vi "Oil_Refinery.vi"() -> ()   [LabVIEW 2024]
uses:
  <vilib>/addons/control/pid/pid.llb/PID (DBL).vi
  <vilib>/addons/control/pid/NI_PID_pid.lvlib
panel:
  out "POWER (W)":dbl(knob) scale=0.0..100000.0 scale format="%#.2f"
  out "U_OUT":dbl(knob) scale=0.0..10000.0
  out "U_IN":dbl(knob) scale=0.0..120000.0
  out "Transformer_On_Light":bool
  in  "Transformer_On":bool
  out "Res Debit":dbl format="%#.2g"
  out "Dis Debit":dbl format="%#.2g"
  out "Gas Debit":dbl format="%#.2g"
  out "Crude Oil Debit":dbl(knob) scale=0.0..10.0
  out "PressPipe3":bool
  in  "EMPTY\nBOILER":bool
  in  "Graph Monitor":T1(tab)
  out "BOILER TEMPERATURE":dbl(graph)=35.0
  out "PID OUTPUT":dbl(graph)
  out "PID-TEMP TREND":cluster{dbl[], dbl[]}(graph)={[35.0, 35.0, 35.0, 35.0, 35.0, 35.0, 35.0, 35.0, 35.0, 35.0, 35.0, 35.0, 35.0, 35.0, 35.0, 35.0, 35.0, 35.0, 35.0, 35.0, 35.0, 35.0, 35.0, 35.0, 35.0, 35.0, 35.0, 35.0, 35.0, 35.0, 35.0, 35.0, 35.0, 35.0, 35.0, 35.0], [35.0, 35.0, 35.0, 35.0, 35.0, 35.0, 35.0, 35.0, 35.0, 35.0, 35.0, 35.0, 35.0, 35.0, 35.0, 35.0, 35.0, 35.0, 35.0, 35.0, 35.0, 35.0, 35.0, 35.0, 35.0, 35.0, 35.0, 35.0, 35.0, 35.0, 35.0, 35.0, 35.0, 35.0, 35.0, 35.0]}
  in  "PID gains":T2={"proportional gain (Kc)"=2.0, "integral time (Ti, min)"=0.05, "derivative time (Td, min)"=0.1}
  in  "HEATER POWER":u64(knob) scale=0.0..10.0
  out "PID output":dbl format="%.2f"
  out "PID %":dbl(slide)=35.0 scale=0.0..100.0 scale format="%#.2g"
  out "BAR":dbl(knob)=0.8301077246178509 scale=0.0..100.0
  out "HEATER":bool
  out "BOILER TEMP":dbl(knob)=35.0 scale=0.0..800.0
  out "RESIDUE":dbl(slide) scale=0.0..100.0
  out "DIESEL":dbl(slide) scale=0.0..100.0
  out "GASOLINE":dbl(slide) scale=0.0..100.0
  out "BOILER":dbl(slide) scale=0.0..100.0
  in  "Setpoint °C":dbl(knob)=100.0 scale=100.0..800.0
  in  "EMPTY\nCRUDE\nOIL \nTANK":bool
  out "Boiler Level":dbl(knob) scale=0.0..100.0 scale format="%#.2g"
  out "?":bool
  in  "Refill\nCrude Oil\nTank":bool
  out "Crude Oil Level":dbl(knob) scale=0.0..100.0 scale format="%#.2g"
  out "?":bool
  out "?":bool
  out "?":bool
  out "?":bool
  out "?":bool
  out "?":bool
  out "?":bool
  in  "Over\nPressure\nValve":bool
  in  "OIL PUMP":bool
  in  "Residue \nValve":bool
  in  "Diesel\nValve":bool
  in  "Gasoline Valve":bool
  in  "Crude \nOil\nValve":bool
  in  "STOP SIM":bool
  in  "HEATER":bool
  out "GaspolinePipe2":bool
  out "DieselPipe2":bool
  out "ResiduePipe2":bool
  out "OilPipe2":bool
  out "PressPipe2":bool
  out "PressPipe1":bool
  out "GaspolinePipe1":bool
  out "DieselPipe1":bool
  out "ResiduePipe1":bool
  out "OilPipe3":bool
  out "BOILER PRESSURE":dbl(slide) scale=0.0..100.0
  out "Oil_Pump":bool
  out "OilPipe1":bool
  out "Residue_Valve":bool
  out "Diesel_Valve":bool
  out "Gasoline_Valve":bool
  out "OverPressure_Valve":bool
  out "Crude_Oil_Valve":bool
  out "Alarm and Event Display":refnum<k7>(container)
  in  "Set Crude Oil Level":dbl(slide) scale=0.0..100.0
  out "CRUDE OIL TANK":dbl(slide) scale=0.0..100.0
  # "GREASY DUCK\n OIL PLANT"
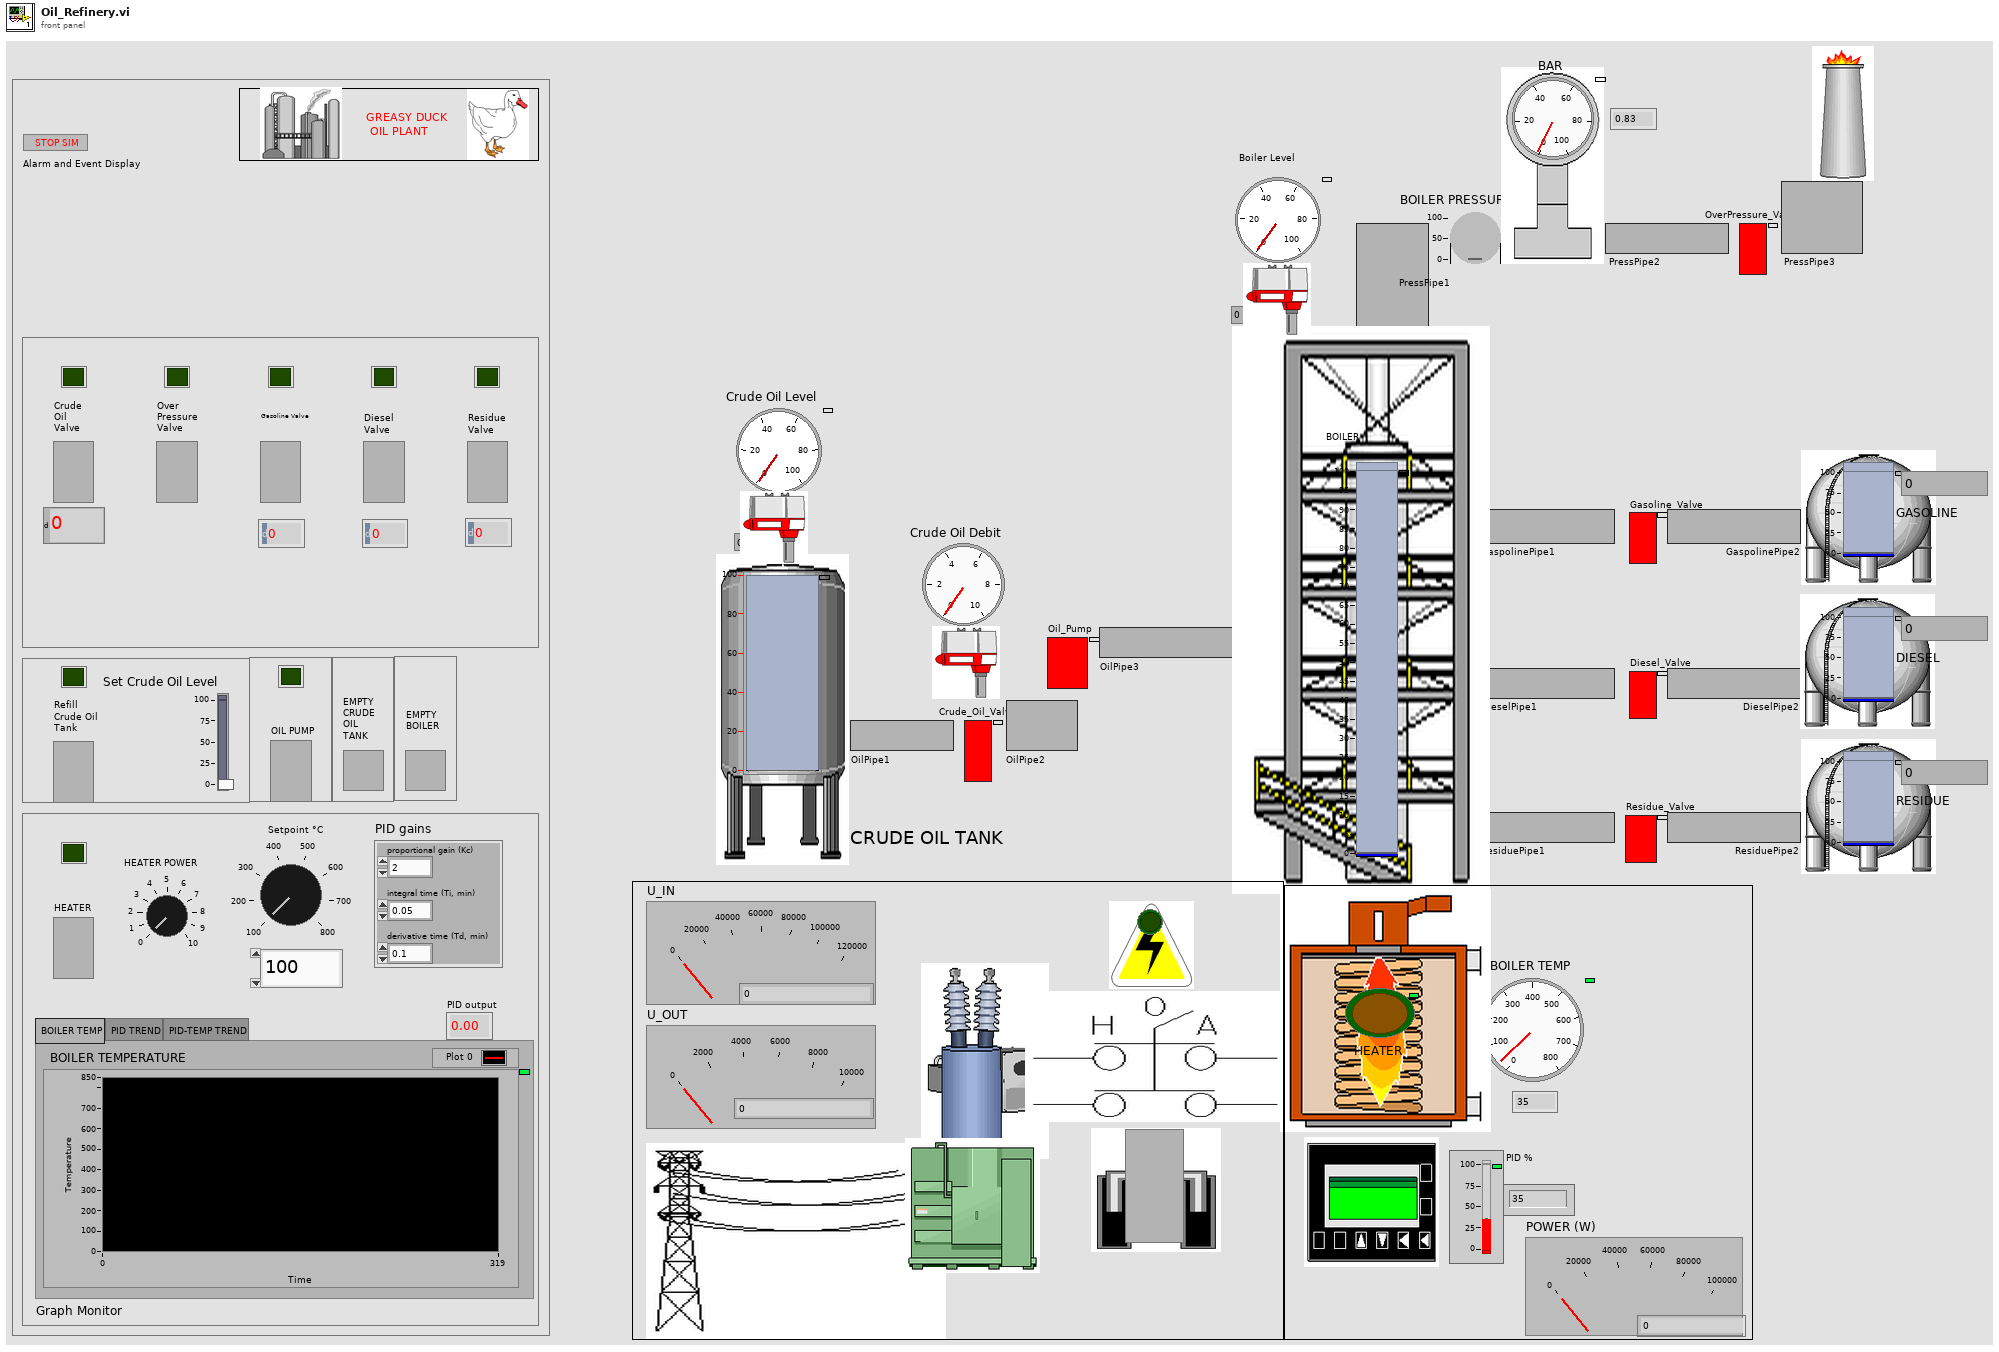
[diagram p1: front panel]
types:
  T1 = enum32{"BOILER TEMP", "PID TREND", "PID-TEMP TREND"}
  T2 = cluster{"proportional gain (Kc)":dbl, "integral time (Ti, min)":dbl, "derivative time (Td, min)":dbl}
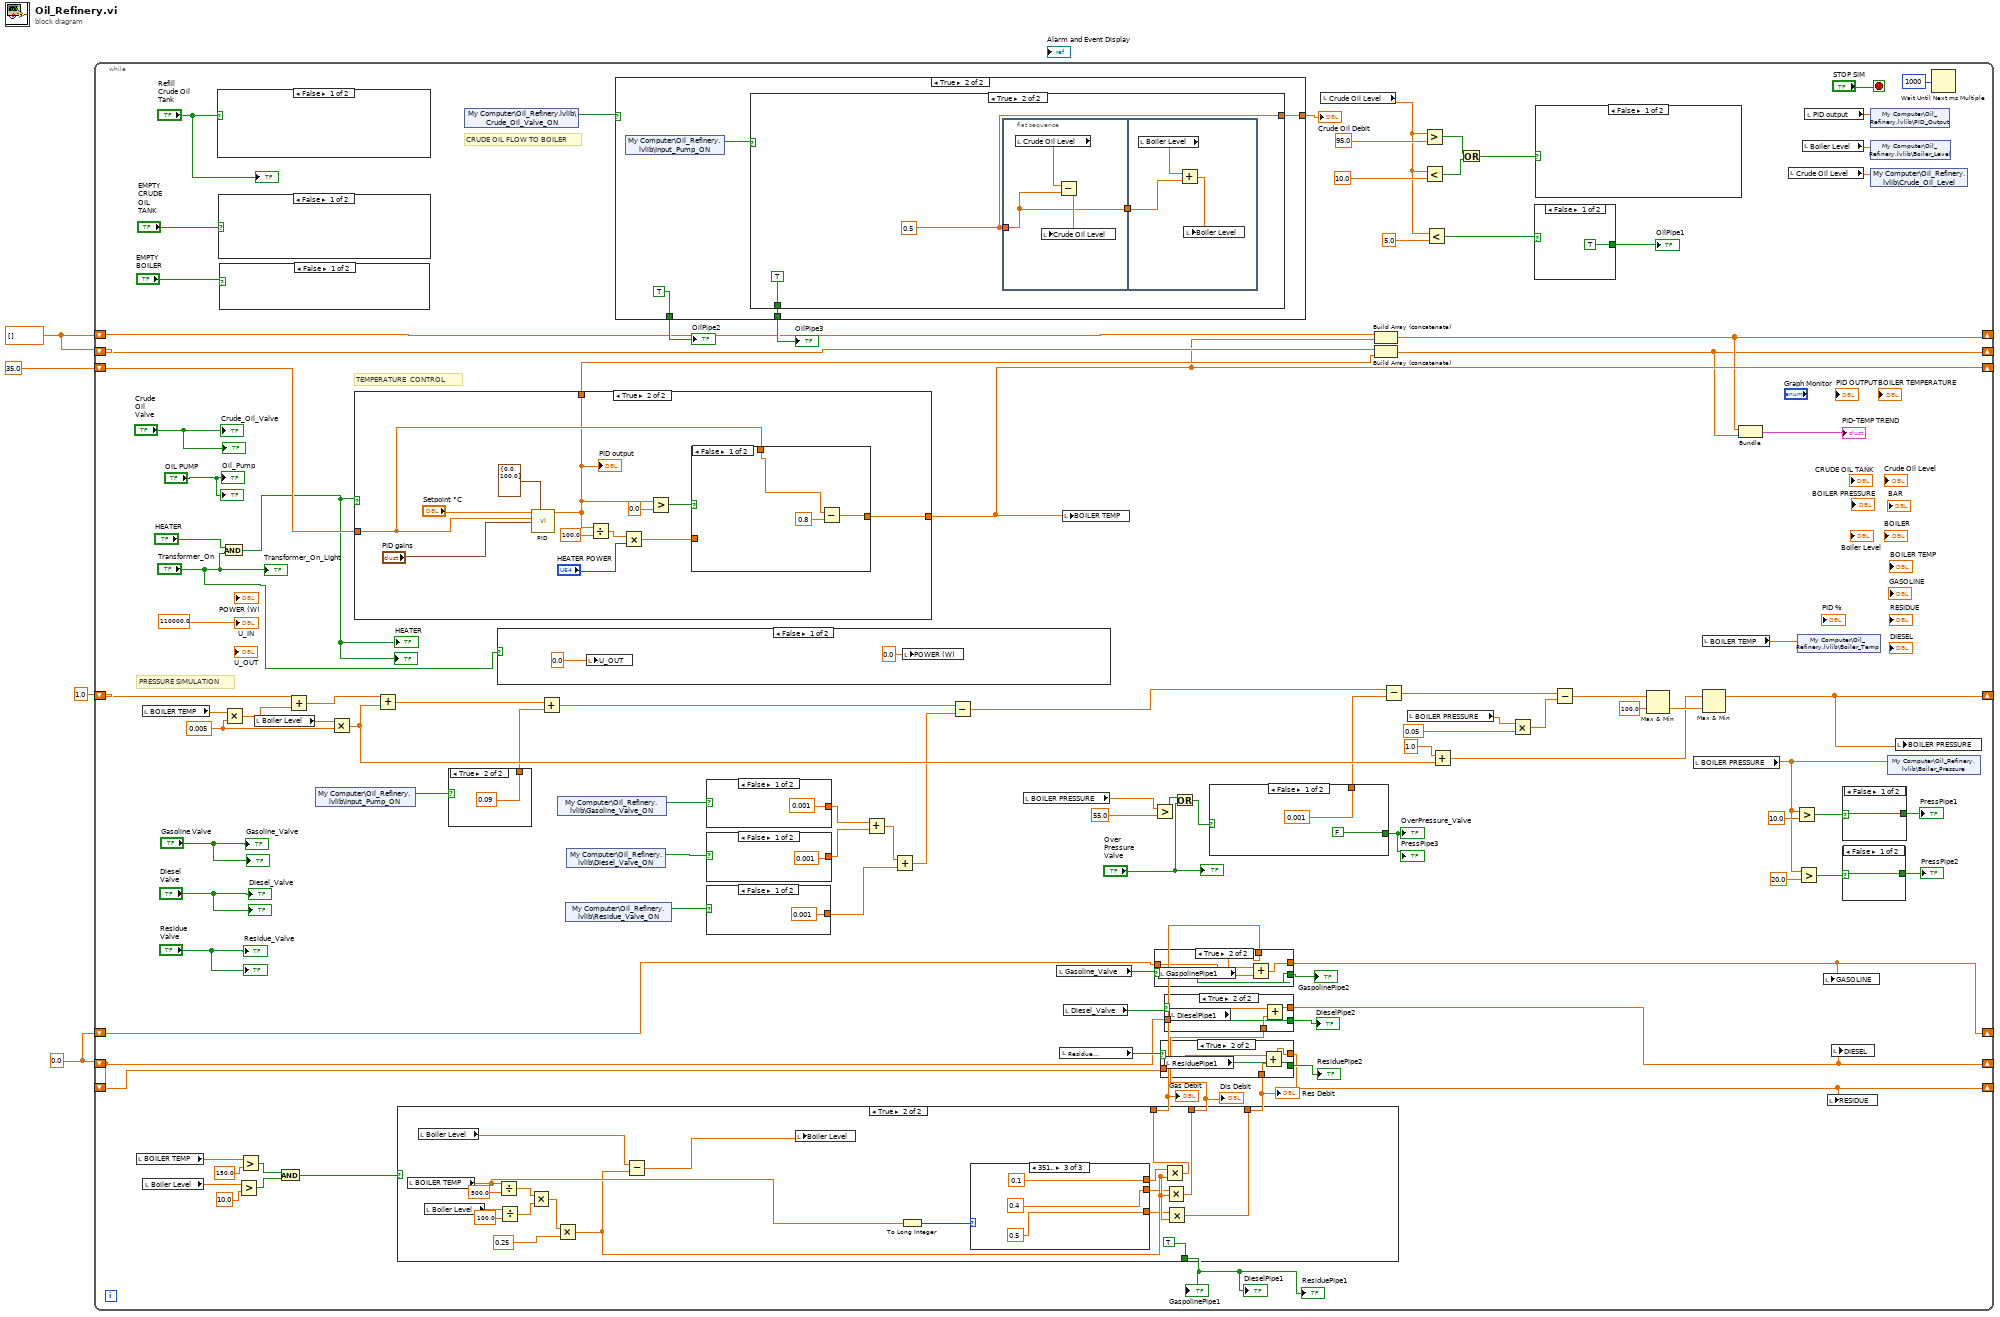
[diagram p0: block diagram]
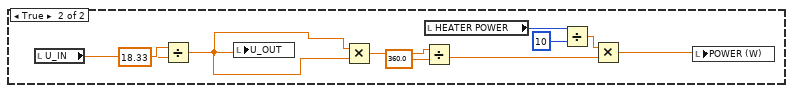
[diagram p2: hidden frame]
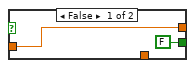
[diagram p3: hidden frame]
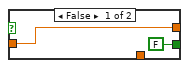
[diagram p4: hidden frame]
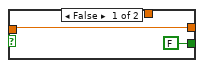
[diagram p5: hidden frame]
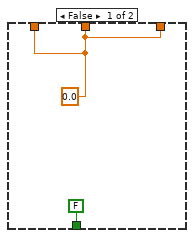
[diagram p6: hidden frame]
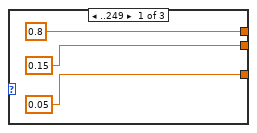
[diagram p7: hidden frame]
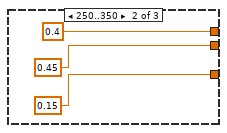
[diagram p8: hidden frame]
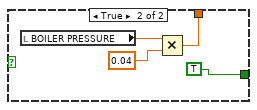
[diagram p11: hidden frame]
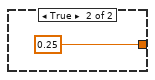
[diagram p12: hidden frame]
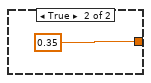
[diagram p13: hidden frame]
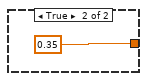
[diagram p14: hidden frame]
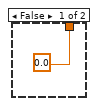
[diagram p15: hidden frame]
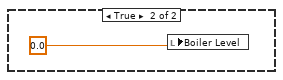
[diagram p16: hidden frame]
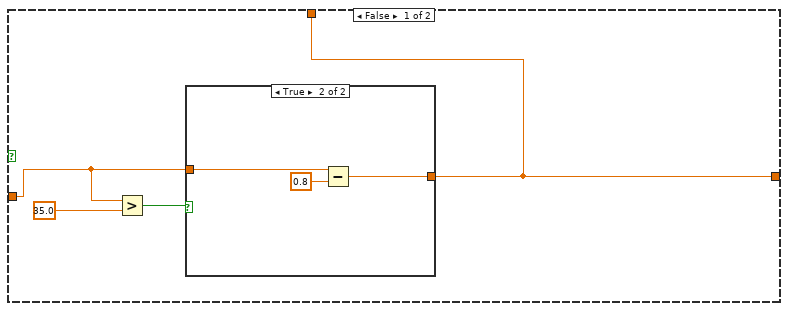
[diagram p17: hidden frame]
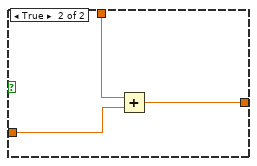
[diagram p19: hidden frame]
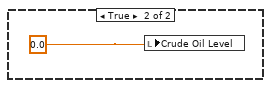
[diagram p20: hidden frame]
diagram:
  w1 = 0.0
  w3 = dbl[] []
  n1 = while {
    shift-right: [w82] -> _
    shift-left: 35.0 -> [w88]
    shift-right: [w80] -> _
    shift-left: w3 -> [w85]
    shift-right: [w79] -> _
    shift-left: w3 -> [w84]
    shift-right: [w71] -> _
    shift-left: 1.0 -> [w76]
    shift-right: [w10] -> _
    shift-left: w1 -> [w13]
    shift-right: [w11] -> _
    shift-left: w1 -> [w18]
    shift-right: [w12] -> _
    shift-left: w1 -> [w17]
    stop <- "STOP SIM" stop-if-true
    w65 = 0.005
    # "CRUDE OIL FLOW TO BOILER"
    # "TEMPERATURE  CONTROL"
    # "PRESSURE SIMULATION"
    n2 = local read "BOILER TEMP"() -> (w32:dbl)
    n3 = local read "BOILER TEMP"() -> (w74:dbl)
    n4 = local read "Boiler Level"() -> (w31:dbl)
    n5 = case shown="False" "Refill\nCrude Oil\nTank" {
      frame False {
      }
      frame True {
        n6 = local write "Crude Oil Level"("Set Crude Oil Level") -> ()
      }
    }
    n7 = case shown="False" "EMPTY\nCRUDE\nOIL \nTANK" {
      frame False {
      }
      frame True {
        n8 = local write "Crude Oil Level"(0.0) -> ()
      }
    }
    n9 = case shown="False" "EMPTY\nBOILER" {
      frame False {
      }
      frame True {
        n10 = local write "Boiler Level"(0.0) -> ()
      }
    }
    n11 = And(x="HEATER", y="Transformer_On") -> (x .and. y?=w7:bool)
    "?" <- w7
    "HEATER" <- w7
    n12 = Multiply(x=w74, y=w65) -> (x*y=w75:dbl)
    n13 = Greater?(x=w31, y=10.0) -> (0:w27:bool)
    n14 = Greater?(x=w32, y=150.0) -> (0:w28:bool)
    n15 = local read "Boiler Level"() -> (w64:dbl)
    n16 = And(x=w28, y=w27) -> (x .and. y?=w26:bool)
    n17 = Add(x=w76, y=w75) -> (x+y=w66:dbl)
    n18 = shared-variable "My Computer\\Oil_Refinery.lvlib\\Input_Pump_ON"() -> (w60:bool)  [unwired: 1 in, 1 out]
    n19 = Multiply(x=w64, y=w65) -> (x*y=w61:dbl)
    n20 = case shown="True" w7 {
      tunnel: w88 -> [w192 w201]
      tunnel: [w190 w203] -> w82
      tunnel: [w190 w198] -> w83
      frame False {
        n21 = Greater?(x=w192, y=35.0) -> (0:w193:bool)
        n22 = case shown="True" w193 {
          tunnel: [w194 w197] -> w190
          tunnel: w192 -> [w194 w196]
          frame False {
          }
          frame True {
            n23 = Subtract(x=w196, y=0.8) -> (x-y=w197:dbl)
          }
        }
      }
      frame True {
        n24 = call-poly <vilib>:"PID.vi"("output range"=cluster{"output high":dbl, "output low":dbl} {"output high"=0.0, "output low"=100.0}, "PID gains"="PID gains", "process variable"=w201, "setpoint"="Setpoint °C") -> ("output"=w198:dbl)  [unwired: 6 in, 1 out]
        "PID output" <- w198
        n25 = Divide(x=w198, y=100.0) -> (x/y=w205:dbl)
        n26 = Multiply(x=w205, y="HEATER POWER") -> (x*y=w202:dbl)
        n27 = Greater?(x=w198, y=0.0) -> (0:w200:bool)
        n28 = case shown="False" w200 {
          tunnel: [w211 w215] -> w203
          tunnel: w202 -> [_ w214]
          tunnel: w201 -> [w210 w213]
          frame False {
            n29 = Subtract(x=w210, y=0.8) -> (x-y=w211:dbl)
          }
          frame True {
            n30 = Add(x=w213, y=w214) -> (x+y=w215:dbl)
          }
        }
      }
    }
    n31 = Add(x=w66, y=w61) -> (x+y=w59:dbl)
    n32 = case shown="True" w26 {
      tunnel: [FALSE TRUE] -> w25
      tunnel: [w141 w145] -> w16
      tunnel: [w141 w144] -> w15
      tunnel: [w141 w143] -> w14
      frame False {
        w141 = 0.0
      }
      frame True {
        n33 = local read "BOILER TEMP"() -> (w151:dbl)
        n34 = local read "Boiler Level"() -> (w154:dbl)
        n35 = local read "Boiler Level"() -> (w160:dbl)
        n36 = Divide(x=w151, y=500.0) -> (x/y=w158:dbl)
        n37 = Divide(x=w160, y=100.0) -> (x/y=w157:dbl)
        n38 = Multiply(x=w158, y=w157) -> (x*y=w156:dbl)
        n39 = Multiply(x=w156, y=0.25) -> (x*y=w149:dbl)
        n40 = Subtract(x=w154, y=w149) -> (x-y=w153:dbl)
        n41 = local write "Boiler Level"(w153) -> ()
        n42 = To Long Integer(number=w151) -> (32bit integer=w152:i32)
        n43 = case shown="351.." w152 {
          tunnel: [0.8 0.4 0.1] -> w148
          tunnel: [0.15 0.45 0.4] -> w147
          tunnel: [0.05 0.15 0.5] -> w146
          frame ..249 {
          }
          frame 250..350 {
          }
          frame 351.. {
          }
        }
        n44 = Multiply(x=w148, y=w149) -> (x*y=w145:dbl)
        n45 = Multiply(x=w147, y=w149) -> (x*y=w144:dbl)
        n46 = Multiply(x=w146, y=w149) -> (x*y=w143:dbl)
      }
    }
    "GaspolinePipe1" <- w25
    "DieselPipe1" <- w25
    "ResiduePipe1" <- w25
    "Gas Debit" <- w16
    "Dis Debit" <- w15
    "Res Debit" <- w14
    n47 = case shown="True" w60 {
      tunnel: [0.0 0.09] -> w58
      frame False {
      }
      frame True {
      }
    }
    n48 = shared-variable "My Computer\\Oil_Refinery.lvlib\\Crude_Oil_Valve_ON"() -> (w106:bool)  [unwired: 1 in, 1 out]
    n49 = case shown="False" "Transformer_On" {
      frame False {
        n50 = local write "U_OUT"(0.0) -> ()
        n51 = local write "POWER (W)"(0.0 ("POWER (W)")) -> ()
      }
      frame True {
        n52 = local read "U_IN"() -> (w122:dbl)
        n53 = Divide(x=w122, y=18.33) -> (x/y=w120:dbl)
        n54 = local write "U_OUT"(w120) -> ()
        n55 = Multiply(x=w120, y=w120) -> (x*y=w117:dbl)
        n56 = Divide(x=w117, y=360.0) -> (x/y=w113:dbl)
        n57 = local read "HEATER POWER"() -> (w119:u64)
        n58 = Divide(x=w119, y=u64 10) -> (x/y=w115:dbl)
        n59 = Multiply(x=w115, y=w113) -> (x*y=w114:dbl)
        n60 = local write "POWER (W)"(w114) -> ()
      }
    }
    n61 = Add(x=w59, y=w58) -> (x+y=w50:dbl)
    n62 = shared-variable "My Computer\\Oil_Refinery.lvlib\\Gasoline_Valve_ON"() -> (w55:bool)  [unwired: 1 in, 1 out]
    n63 = shared-variable "My Computer\\Oil_Refinery.lvlib\\Residue_Valve_ON"() -> (w57:bool)  [unwired: 1 in, 1 out]
    n64 = shared-variable "My Computer\\Oil_Refinery.lvlib\\Diesel_Valve_ON"() -> (w56:bool)  [unwired: 1 in, 1 out]
    n65 = case shown="True" w106 {
      tunnel: [FALSE TRUE] -> w105
      tunnel: [FALSE w226] -> w104
      tunnel: [0.0 w224] -> w9
      frame False {
      }
      frame True {
        n66 = shared-variable "My Computer\\Oil_Refinery.lvlib\\Input_Pump_ON"() -> (w227:bool)  [unwired: 1 in, 1 out]
        n67 = case shown="True" w227 {
          tunnel: [FALSE TRUE] -> w226
          tunnel: [0.0 w230] -> w224
          frame False {
          }
          frame True {
            w230 = 0.5 ("y")
            n68 = flat-sequence {
              tunnel: w230 -> [w233]
              tunnel: [w233] -> w231
              tunnel: w231 -> [w236]
              frame #0 {
                n69 = local read "Crude Oil Level"() -> (w235:dbl)
                n70 = Subtract(x=w235, y=w233) -> (x-y=w234:dbl)
                n71 = local write "Crude Oil Level"(w234) -> ()
              }
              frame #1 {
                n72 = local read "Boiler Level"() -> (w237:dbl)
                n73 = Add(x=w237, y=w236) -> (x+y=w238:dbl)
                n74 = local write "Boiler Level"(w238) -> ()
              }
            }
          }
        }
      }
    }
    "OilPipe3" <- w104
    "OilPipe2" <- w105
    "Crude Oil Debit" <- w9
    n75 = case shown="False" w57 {
      tunnel: [0.001 0.25] -> w51
      frame False {
      }
      frame True {
      }
    }
    n76 = case shown="False" w55 {
      tunnel: [0.001 0.35] -> w54
      frame False {
      }
      frame True {
      }
    }
    n77 = case shown="False" w56 {
      tunnel: [0.001 0.35] -> w53
      frame False {
      }
      frame True {
      }
    }
    n78 = Add(x=w54, y=w53) -> (x+y=w52:dbl)
    n79 = Add(x=w52, y=w51) -> (x+y=w49:dbl)
    n80 = Subtract(x=w50, y=w49) -> (x-y=w43:dbl)
    n81 = local read "BOILER PRESSURE"() -> (w48:dbl)
    n82 = local read "Gasoline_Valve"() -> (w21:bool)
    n83 = local read "Residue \nValve"() -> (w19:bool)
    n84 = local write "BOILER TEMP"(w82) -> ()
    n85 = local read "Diesel_Valve"() -> (w20:bool)
    n86 = Greater?(x=w48, y=55.0) -> (0:w46:bool)
    n87 = case shown="True" w21 {
      tunnel: [FALSE w137] -> w24
      tunnel: [w135 w139] -> w10
      tunnel: w16 -> [_ w140]
      tunnel: w13 -> [w135 w138]
      frame False {
      }
      frame True {
        n88 = local read "GaspolinePipe1"() -> (w137:bool)
        n89 = Add(x=w138, y=w140) -> (x+y=w139:dbl)
      }
    }
    "GaspolinePipe2" <- w24
    n90 = case shown="True" w19 {
      tunnel: [FALSE w125] -> w22
      tunnel: w17 -> [w123 w128]
      tunnel: [w123 w127] -> w12
      tunnel: w14 -> [_ w126]
      frame False {
      }
      frame True {
        n91 = local read "ResiduePipe1"() -> (w125:bool)
        n92 = Add(x=w128, y=w126) -> (x+y=w127:dbl)
      }
    }
    "ResiduePipe2" <- w22
    n93 = case shown="True" w20 {
      tunnel: [FALSE w131] -> w23
      tunnel: w18 -> [w129 w134]
      tunnel: [w129 w133] -> w11
      tunnel: w15 -> [_ w132]
      frame False {
      }
      frame True {
        n94 = local read "DieselPipe1"() -> (w131:bool)
        n95 = Add(x=w134, y=w132) -> (x+y=w133:dbl)
      }
    }
    "DieselPipe2" <- w23
    n96 = Or(x=w46, y="Over\nPressure\nValve") -> (x .or. y?=w41:bool)
    n97 = case shown="False" w41 {
      tunnel: [0.001 w178] -> w42
      tunnel: [FALSE TRUE] -> w40
      frame False {
      }
      frame True {
        n98 = local read "BOILER PRESSURE"() -> (w180:dbl)
        n99 = Multiply(x=w180, y=0.04) -> (x*y=w178:dbl)
      }
    }
    "OverPressure_Valve" <- w40
    "PressPipe3" <- w40
    n100 = local read "Crude Oil Level"() -> (w92:dbl)
    n101 = Build Array (concatenate)(w85, w82) -> (w80:dbl[])
    n102 = Build Array (concatenate)(w84, w83) -> (w79:dbl[])
    n103 = Subtract(x=w43, y=w42) -> (x-y=w44:dbl)
    n104 = local read "BOILER PRESSURE"() -> (w69:dbl)
    n105 = Greater?(x=w92, y=95.0) -> (0:w102:bool)
    n106 = Less?(x=w92, y=10.0) -> (x < y?=w101:bool)
    n107 = Less?(x=w92, y=5.0) -> (x < y?=w97:bool)
    n108 = Add(x=1.0, y=w61) -> (x+y=w62:dbl)
    n109 = Or(x=w102, y=w101) -> (x .or. y?=w103:bool)
    n110 = Multiply(x=w69, y=0.05) -> (x*y=w67:dbl)
    n111 = case shown="False" w97 {
      tunnel: [TRUE ("OilPipe1") FALSE ("OilPipe1")] -> w98
      frame False {
      }
      frame True {
      }
    }
    "OilPipe1" <- w98
    n112 = case shown="False" w103 {
      frame False {
      }
      frame True {
        w220 = FALSE
        n113 = shared-variable "My Computer\\Oil_Refinery.lvlib\\Crude_Oil_Valve_ON"(w220) -> ()  [unwired: 1 in, 1 out]
        n114 = shared-variable "My Computer\\Oil_Refinery.lvlib\\Input_Pump_ON"(w220) -> ()  [unwired: 1 in, 1 out]
      }
    }
    n115 = Subtract(x=w44, y=w67) -> (x-y=w70:dbl)
    n116 = Max & Min(x=w70, y=100.0) -> (min(x,y)=w72:dbl)  [unwired: 1 out]
    n117 = local read "BOILER PRESSURE"() -> (w33:dbl)
    n118 = local read "BOILER TEMP"() -> (w87:dbl)
    n119 = Max & Min(x=w62, y=w72) -> (max(x,y)=w71:dbl)  [unwired: 1 out]
    n120 = Bundle(w80, w79) -> (→"PID-TEMP TREND":cluster{dbl[], dbl[]})  [unwired: 1 in]
    n121 = local read "Crude Oil Level"() -> (w90:dbl)
    n122 = Greater?(x=w33, y=10.0) -> (0:w37:bool)
    n123 = shared-variable "My Computer\\Oil_Refinery.lvlib\\Boiler_Temp"(w87) -> ()  [unwired: 1 in, 1 out]
    n124 = Greater?(x=w33, y=20.0) -> (0:w36:bool)
    n125 = local read "Boiler Level"() -> (w91:dbl)
    n126 = local read "PID output"() -> (w86:dbl)
    n127 = local write "GASOLINE"(w10) -> ()
    n128 = local write "RESIDUE"(w12) -> ()
    n129 = local write "DIESEL"(w11) -> ()
    n130 = case shown="False" w37 {
      selector: w37 -> [w173 w174]
      tunnel: [w173 w174] -> w38
      frame False {
      }
      frame True {
      }
    }
    "PressPipe1" <- w38
    n131 = case shown="False" w36 {
      selector: w36 -> [w171 w172]
      tunnel: [w171 w172] -> w39
      frame False {
      }
      frame True {
      }
    }
    "PressPipe2" <- w39
    n132 = shared-variable "My Computer\\Oil_Refinery.lvlib\\PID_Output"(w86) -> ()  [unwired: 1 in, 1 out]
    n133 = shared-variable "My Computer\\Oil_Refinery.lvlib\\Boiler_Level"(w91) -> ()  [unwired: 1 in, 1 out]
    n134 = shared-variable "My Computer\\Oil_Refinery.lvlib\\Crude_Oil_Level"(w90) -> ()  [unwired: 1 in, 1 out]
    n135 = shared-variable "My Computer\\Oil_Refinery.lvlib\\Boiler_Pressure"(w33) -> ()  [unwired: 1 in, 1 out]
    n136 = local write "BOILER PRESSURE"(w71) -> ()
    n137 = Wait Until Next ms Multiple(millisecond multiple=u32 1000) -> ()  [unwired: 1 out]
    "?" <- "Crude \nOil\nValve"
    "?" <- "OIL PUMP"
    "?" <- "Over\nPressure\nValve"
    "?" <- "Gasoline Valve"
    "?" <- "Diesel\nValve"
    "?" <- "Residue \nValve"
    "Crude_Oil_Valve" <- "Crude \nOil\nValve"
    "Oil_Pump" <- "OIL PUMP"
    "Gasoline_Valve" <- "Gasoline Valve"
    "Diesel_Valve" <- "Diesel\nValve"
    "Residue_Valve" <- "Residue \nValve"
    "?" <- "Refill\nCrude Oil\nTank"
    "Transformer_On_Light" <- "Transformer_On"
    "U_IN" <- 110000.0 ("x")
  }
